vi "Create Dev Panel.vi"(10 "Dev Panel":refnum<class "Dev Panel.lvclass">, 11 "Dev Actor in":refnum<class "Dev Actor.lvclass">) -> (0 "error out":errorcluster, 3 "Dev Actor out":refnum<class "Dev Actor.lvclass">)   [LabVIEW 2021, in "Dev Actor.lvlib" / "Dev Actor.lvclass"]
uses:
  Dev Actor.lvclass
  Dev Panel/Dev Panel.lvclass
  C:/git/jettl/src/Event Actor/Event Actor.lvclass
  Dev Actor.lvclass/Dev Actor.ctl
  Actor/Event Actor/Event Actor.lvclass
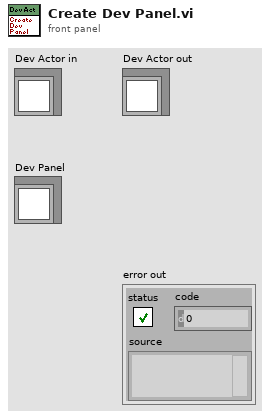
[diagram p1: front panel]
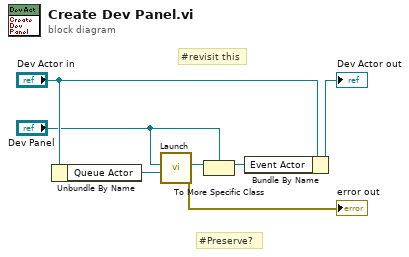
[diagram p0: block diagram]
diagram:
  # "#revisit this"
  # "#Preserve?"
  n1 = Unbundle By Name("Dev Actor in") -> ("Queue Actor"=w2:refnum<class "Queue Actor.lvclass">)
  n2 = call "Launch.vi"("Queue Actor"=w2, "Event Actor"="Dev Panel") -> ("error out"=→"error out":errorcluster, "Event Actor"=w3:refnum<class "Event Actor.lvclass">)  [unwired: 8 in]
  n3 = To More Specific Class(target class="Dev Panel", reference=w3) -> (specific class reference=w5:refnum<class "Dev Panel.lvclass">)  [unwired: 1 in, 1 out]
  n4 = Bundle By Name(cluster="Dev Actor in", "Event Actor"=w5) -> (→"Dev Actor out":refnum<class "Dev Actor.lvclass">)
